vi "Set Environment Variable.vi"(7 "Target (Process)":T1 items=["Process", "User", "Machine"], 8 "Error In":errorcluster, 10 "Value":string, 11 "Name":string) -> (0 "Error Out":errorcluster)   [LabVIEW 2019, in "SLL Environment Variable.lvlib"]
doc: "Set <B>Value</B> to the environment variable in the <B>Target</B> environment."
uses:
  SLL Environment Variable.lvlib
  _Typedef/Target Environment Enum.ctl
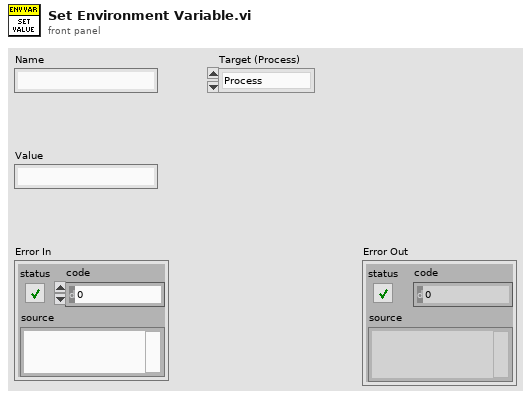
[diagram p1: front panel]
types:
  T1 = typedef "SLL Environment Variable.lvlib/Target Environment Enum.ctl" = i32
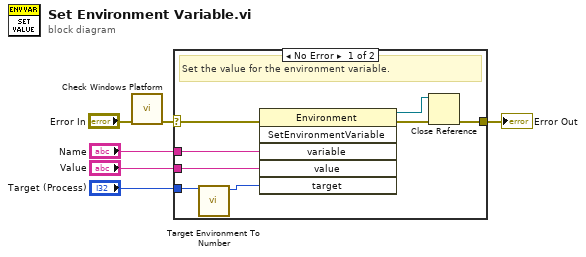
[diagram p0: block diagram]
diagram:
  n1 = call "Check Windows Platform.vi"("Error In"="Error In") -> ("Error Out"=w2:errorcluster)  [unwired: 10 in]
  n2 = case shown="No Error" w2 {
    selector: w2 -> [w14 w15]
    tunnel: "Name" -> [w13 _]
    tunnel: [w11 w15] -> w5
    tunnel: "Value" -> [w9 _]
    tunnel: "Target (Process)" -> [w8 _]
    frame No Error {
      # "Set the value for the environment variable."
      n3 = call "Target Environment To Number.vi"("Target (Process)"=w8) -> ("Numeric Value"=w7:i32)  [unwired: 10 in]
      n4 = invoke class="Environment" method="SetEnvironmentVariable"(error in=w14, "variable"=w13, "value"=w9, "target"=w7) -> (reference out=w10:refnum<k24>, error out=w12:errorcluster)  [unwired: 2 in, 4 out]
      n5 = Close Reference(reference=w10, error in (no error)=w12) -> (error out=w11:errorcluster)
    }
    frame Error {
    }
  }
  "Error Out" <- w5
